vi "ILCDisabledTest.vi"() -> ()   [LabVIEW 2016]
uses:
  Common_RT_HPILC/DataTypes/HPTelemetry.ctl
  Stats.ctl
  Common_RT_Modbus/DataTypes/RxFrame.ctl
  Common_RT_HealthAndStatus/RTHealthAndStatus/RTHealthAndStatus.lvclass
  MyHealthAndStatusReadFIFO/MyHealthAndStatusReadFIFO.lvclass
  D:/Code/Common_RT_FPGA/IReadU32FIFO/IReadU32FIFO.lvclass
  MyHealthAndStatusWriteFIFO/MyHealthAndStatusWriteFIFO.lvclass
  D:/Code/Common_RT_FPGA/IWriteU64FIFO/IWriteU64FIFO.lvclass
  ModbusFactory/ModbusFactory.lvclass
  D:/Code/Common_RT_Modbus/IModbusFactory/IModbusFactory.lvclass
  SubnetFactory/SubnetFactory.lvclass
  Subnet/DataTypes/SubnetSettings.ctl
  Common_RT_HPILC/DataTypes/HPSettings.ctl
  Common_RT_ILC/DataTypes/ILCSettings.ctl
  Common_RT_Modbus/IModbusFactory/IModbusFactory.lvclass
  Common_RT_MTILC/DataTypes/MTSettings.ctl
  Common_RT_MDILC/DataTypes/MDSettings.ctl
  Common_RT_MIILC/DataTypes/MISettings.ctl
  ModbusFactory/ModbusFactory.lvclass/ModbusFactory.ctl
  MyHealthAndStatusWriteFIFO/MyHealthAndStatusWriteFIFO.lvclass/MyHealthAndStatusWriteFIFO.ctl
  MyHealthAndStatusReadFIFO/MyHealthAndStatusReadFIFO.lvclass/MyHealthAndStatusReadFIFO.ctl
  Common_RT_HealthAndStatus/RTHealthAndStatus/RTHealthAndStatus.lvclass/RTHealthAndStatus.ctl
  Subnet/Subnet.lvclass/Subnet.ctl
  Common_RT_HPILC/HPILC/HPILC.lvclass/HPILC.ctl
  <vilib>/Platform/TimedLoop/XDataNode/timing_clust.ctl
  <vilib>/Platform/TimedLoop/XDataNode/nitl_modes.ctl
  <vilib>/Platform/TimedLoop/XDataNode/wakeup.ctl
  Common_RT_MIILC/MIILC/MIILC.lvclass/MIILC.ctl
  Common_RT_MDILC/MDILC/MDILC.lvclass/MDILC.ctl
  Common_RT_MTILC/MTILC/MTILC.lvclass/MTILC.ctl
  <vilib>/FPGAPlugInAG/cRIO-9038/niLvFpga_Open_cRIO-9038.vi
  <vilib>/rvi/interface/common/dynamic/niFpgaDynamicAddResources.vi
  <vilib>/FPGAPlugInAG/Dynamic/niLvFpga_Abort_Dynamic.vi
  <vilib>/FPGAPlugInAG/Dynamic/niLvFpga_Reset_Dynamic.vi
  <vilib>/FPGAPlugInAG/Dynamic/niLvFpga_Run_Dynamic.vi
  <vilib>/Utility/error.llb/Error Cluster From Error Code.vi
  <vilib>/rvi/errors/niLvFpgaAdjustHostInterfaceError.vi
  <vilib>/FPGAPlugInAG/Dynamic/niLvFpga_Close_Dynamic.vi
  <vilib>/rvi/interface/nirviOpenFPGA/nirviOpenFPGA.xnode
  FPGA Bitfiles/modbus1Port.lvbitx
  FPGA/main.vi
  <vilib>/rvi/interface/nirviMethod/nirviMethod.xnode
  <vilib>/Platform/TimedLoop/XDataNode/XDataNode.xnode
  <vilib>/rvi/interface/nirviCloseFPGA/nirviCloseFPGA.xnode
  Subnet/Subnet.lvclass
  Common_RT_ILC/RTILC.lvlib
  Common_RT_HPILC/RTHPILC.lvlib
  Common_RT_HPILC/HPILC/HPILC.lvclass
  <vilib>/rvi/errors/niLvFpgaMergeErrorWithErrorCode.vi
  <vilib>/FPGAPlugInAG/Dynamic/niLvFpga_ReadFifo_Dynamic.vi
  Common_RT_MTILC/MTILC/MTILC.lvclass
  Common_RT_MDILC/MDILC/MDILC.lvclass
  Common_RT_MIILC/MIILC/MIILC.lvclass
  Common_RT_MIILC/RTMIILC.lvlib
  Common_RT_MDILC/RTMDILC.lvlib
  Common_RT_MTILC/RTMTILC.lvlib
  <vilib>/Platform/TimedLoop/XDataNode/XDNodeRunTimeDep.lvlib
  Common_RT_Modbus/RTModbus.lvlib
panel:
  out "Avg Time Delta":dbl
  out "Min Time Delta":i64
  out "Max Time Delta":i64
  out "Timestamp":i64
  out "CRC":T1[](array[typedef]) {"Data" format="%02x"}
  out "Displacement":T2(graph)
  out "Inclination":cluster{"Angle":sgl}(graph)
  out "Temperature":T3(graph)
  out "output cluster":T4={"MinLoopTime"=99999.0, "MaxLoopTime"=-99999.0}
  in  "Steps":i32=1
  out "Loop Time":cluster{u32, "Messages":i32}(graph)
  out "InvalidCRCs":i32
  out "Actuator Telemetry":T5[](array[typedef])
  out "Encoder":T6(graph)
  in  "Stop":bool
  out "Port 1 Status Bits":u64 format="%016b"
  out "error out":errorcluster
  out "Port 1 Frames Received":i64
  out "Port 1 Bytes Received":i64
  out "Port 1 Frames Transmitted":i64
  out "Port 1 Bytes Transmitted":i64
  # "Port 1 = Modbus"
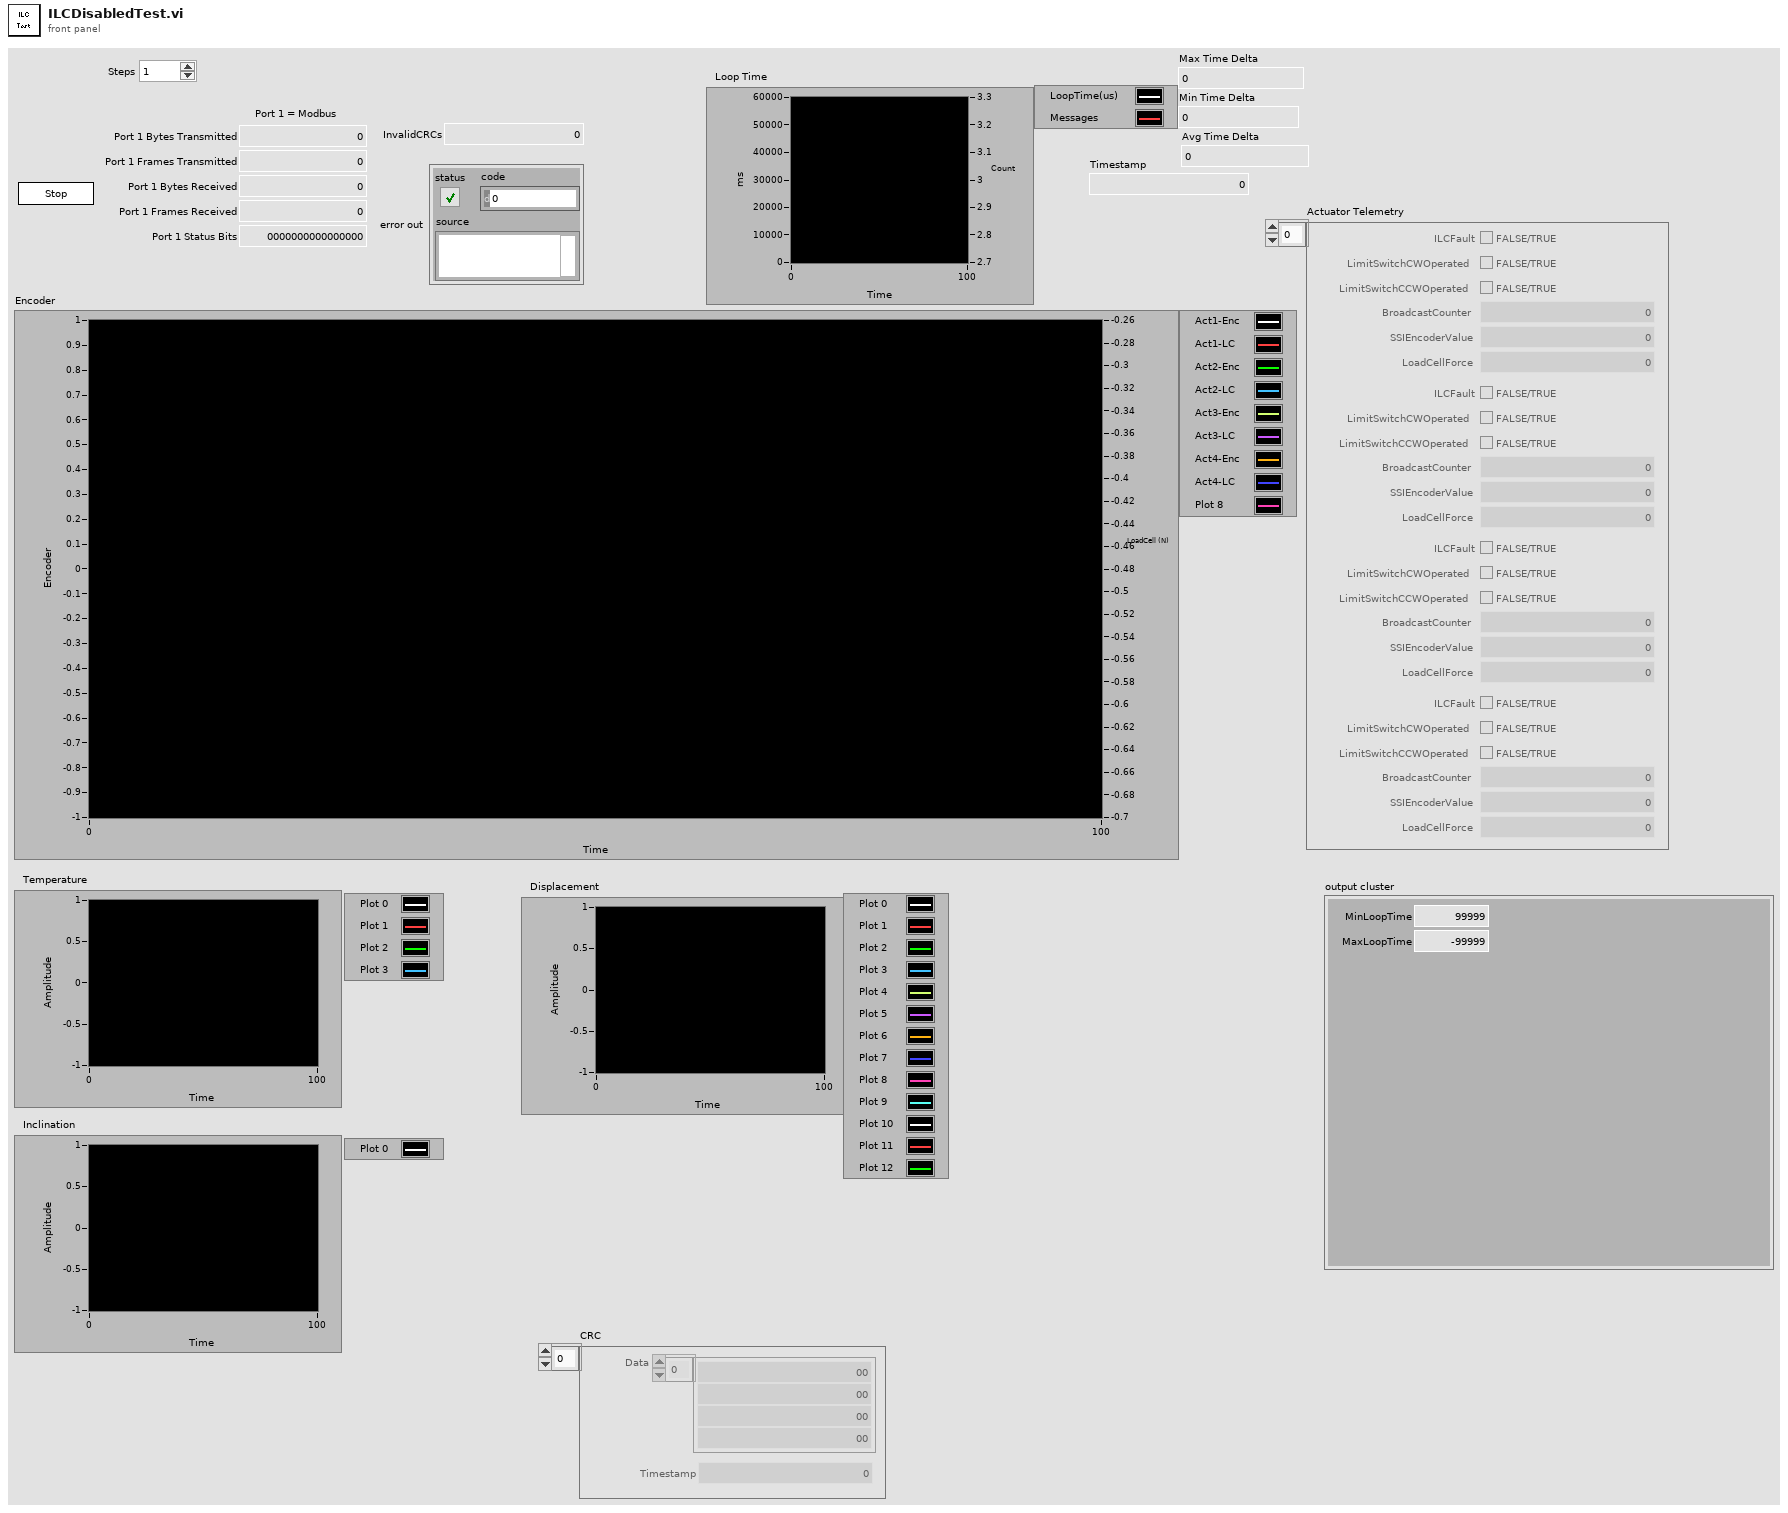
[diagram p1: front panel]
types:
  T1 = typedef "RTModbus.lvlib/RxFrame.ctl" = cluster{"Data":u8[], "Timestamp":u64}
  T2 = cluster{"Displacement1":sgl, "Displacement1":sgl, "Displacement1":sgl, "Displacement1":sgl, "Displacement1":sgl, "Displacement1":sgl}
  T3 = cluster{"Temperature1":sgl, "Temperature1":sgl, "Temperature1":sgl, "Temperature1":sgl}
  T4 = typedef "Stats.ctl" = cluster{"MinLoopTime":dbl, "MaxLoopTime":dbl}
  T5 = typedef "RTHPILC.lvlib/HPTelemetry.ctl" = cluster{"ILCFault":bool, "LimitSwitchCWOperated":bool, "LimitSwitchCCWOperated":bool, "BroadcastCounter":u8, "SSIEncoderValue":i32, "LoadCellForce":sgl}
  T6 = cluster{"[0]":dbl, "[1]":dbl, "[2]":dbl, "[3]":dbl, "[4]":dbl, "[5]":dbl, "[6]":dbl, "[7]":dbl, "[8]":dbl}
  T7 = typedef "RTMIILC.lvlib/MISettings.ctl" = cluster{"ILCSettings":T8, "ID":i16}
  T8 = typedef "RTILC.lvlib/ILCSettings.ctl" = cluster{"Subnet":u8, "Address":u8}
  T9 = typedef "RTMDILC.lvlib/MDSettings.ctl" = cluster{"ILCSettings":T8, "ID":i16}
  T10 = typedef "RTMTILC.lvlib/MTSettings.ctl" = cluster{"ILCSettings":T8, "ID":i16}
  T11 = typedef "RTHPILC.lvlib/HPSettings.ctl" = cluster{"ILCSettings":T8, "ID":i16, "ReferencePosition":i32}
  T12 = enum16{"open", "replace", "create", "open or create", "replace or create", "replace or create with confirmation"}
  T13 = typedef "XDNodeRunTimeDep.lvlib/timing_clust.ctl" = cluster{"Expected End [f-1]":u64, "Actual End [f-1]":u64, "Finished Late? [f-1]":bool, "Expected End [i-1]":u64, "Actual End [i-1]":u64, "Finished Late? [i-1]":bool, "Expected Start [i]":u64, "Actual Start [i]":u64, "Expected Start [f]":u64, "Actual Start [f]":u64, "Source Name":string, "Structure Name":string, "Period":i64, "Deadline":i64, "Offset":i64, "Start":i64, "Priority":i32, "Timeout":i32, "Mode":T14, "Wakeup Reason":T15, "Error":errorcluster, "Source Type":string, "Secondary Source Type":string, "Global End Time":u64, "Global Start Time":u64, "Frame Duration":u64, "Iteration Duration":u64, "Assigned CPU":i32, "I/O Scan Engine Mode":u32}
  T14 = typedef "XDNodeRunTimeDep.lvlib/nitl_modes.ctl" = enum32{"No Change", "Process missed periods, maintain original phase", "Discard missed periods, maintain original phase", "Process missed periods, ignore original phase", "Discard missed periods, ignore original phase"}
  T15 = typedef "XDNodeRunTimeDep.lvlib/wakeup.ctl" = enum32{"Normal", "Aborted", "Asynchronous wakeup", "Timing source error", "Timed loop error", "Timeout"}
  T16 = typedef "SubnetSettings.ctl" = cluster{"HPs":T11[], "ModbusFactory":refnum<class "IModbusFactory.lvclass">, "Port":i32, "MTs":T10[], "MDs":T9[], "MIs":T7[]}
  T17 = typedef "SubnetData.ctl" = cluster{"SubnetConstants":T18, "SubnetCommand":T21, "SubnetTelemetry":T22}
  T18 = typedef "SubnetConstants.ctl" = cluster{"Modbus":refnum<class "IModbus.lvclass">, "HPs":refnum<class "HPILC.lvclass">[], "AddressToActuator":T19[], "MTs":refnum<class "MTILC.lvclass">[], "MDs":refnum<class "MDILC.lvclass">[], "MIs":refnum<class "MIILC.lvclass">[]}
  T19 = typedef "ILCIndexData.ctl" = cluster{"ILCTypes":T20, "Index":i32}
  T20 = typedef "ILCTypes.ctl" = enum16{"Undefined", "SAA", "DAA", "HP", "MT", "MD", "MI"}
  T21 = typedef "SubnetCommand.ctl" = cluster{"BroadcastCounter":u8}
  T22 = typedef "SubnetTelemetry.ctl" = cluster{"BytesTransmitted":u32, "FramesTransmitted":u32, "BytesReceived":u32, "FramesReceived":u32, "TxInternalFIFOOverflow":bool, "InvalidInstruction":bool, "WaitForRxFrameTimeout":bool, "StartBitError":bool, "StopBitError":bool, "RxDataFIFOOverflow":bool}
  T23 = typedef "RTHPILC.lvlib/HPData.ctl" = cluster{"Constants":T24, "Command":T25, "Telemetry":T5, "Responses":T26, "Timings":T28}
  T24 = typedef "RTHPILC.lvlib/HPConstants.ctl" = cluster{"ID":i16, "ReferencePosition":i32}
  T25 = typedef "RTHPILC.lvlib/HPCommand.ctl" = cluster{"Steps":i8}
  T26 = typedef "RTHPILC.lvlib/HPResponses.ctl" = cluster{"StepMotor":T27, "ForceAndStatus":T27}
  T27 = typedef "RTModbus.lvlib/ExceptionCodes.ctl" = u16
  T28 = typedef "RTHPILC.lvlib/HPTimings.ctl" = cluster{"BroadcastStepMotor":u32, "ForceAndStatus":u32, "FreezeSensorValues":u32, "StepMotor":u32}
  T29 = typedef "RTMTILC.lvlib/MTData.ctl" = cluster{"Constants":T30, "Telemetry":T31, "Responses":T32, "Timings":T33}
  T30 = typedef "RTMTILC.lvlib/MTConstants.ctl" = cluster{"ID":i16}
  T31 = typedef "RTMTILC.lvlib/MTTelemetry.ctl" = cluster{"Temperature":sgl[]}
  T32 = typedef "RTMTILC.lvlib/MTResponses.ctl" = cluster{"Temperature":T27}
  T33 = typedef "RTMTILC.lvlib/MTTimings.ctl" = cluster{"Temperature":u32}
  T34 = typedef "RTMDILC.lvlib/MDData.ctl" = cluster{"Constants":T35, "Telemetry":T36, "Responses":T37, "Timings":T38}
  T35 = typedef "RTMDILC.lvlib/MDConstants.ctl" = cluster{"ID":i16}
  T36 = typedef "RTMDILC.lvlib/MDTelemetry.ctl" = cluster{"Displacement":sgl[]}
  T37 = typedef "RTMDILC.lvlib/MDResponses.ctl" = cluster{"Displacement":T27}
  T38 = typedef "RTMDILC.lvlib/MDTimings.ctl" = cluster{"Displacement":u32}
  T39 = typedef "RTMIILC.lvlib/MIData.ctl" = cluster{"Constants":T40, "Telemetry":T41, "Responses":T42, "Timings":T43}
  T40 = typedef "RTMIILC.lvlib/MIConstants.ctl" = cluster{"ID":i16}
  T41 = typedef "RTMIILC.lvlib/MITelemetry.ctl" = cluster{"Angle":sgl}
  T42 = typedef "RTMIILC.lvlib/MIResponses.ctl" = cluster{"Inclination":T27}
  T43 = typedef "RTMIILC.lvlib/MITimings.ctl" = cluster{"Inclination":u32}
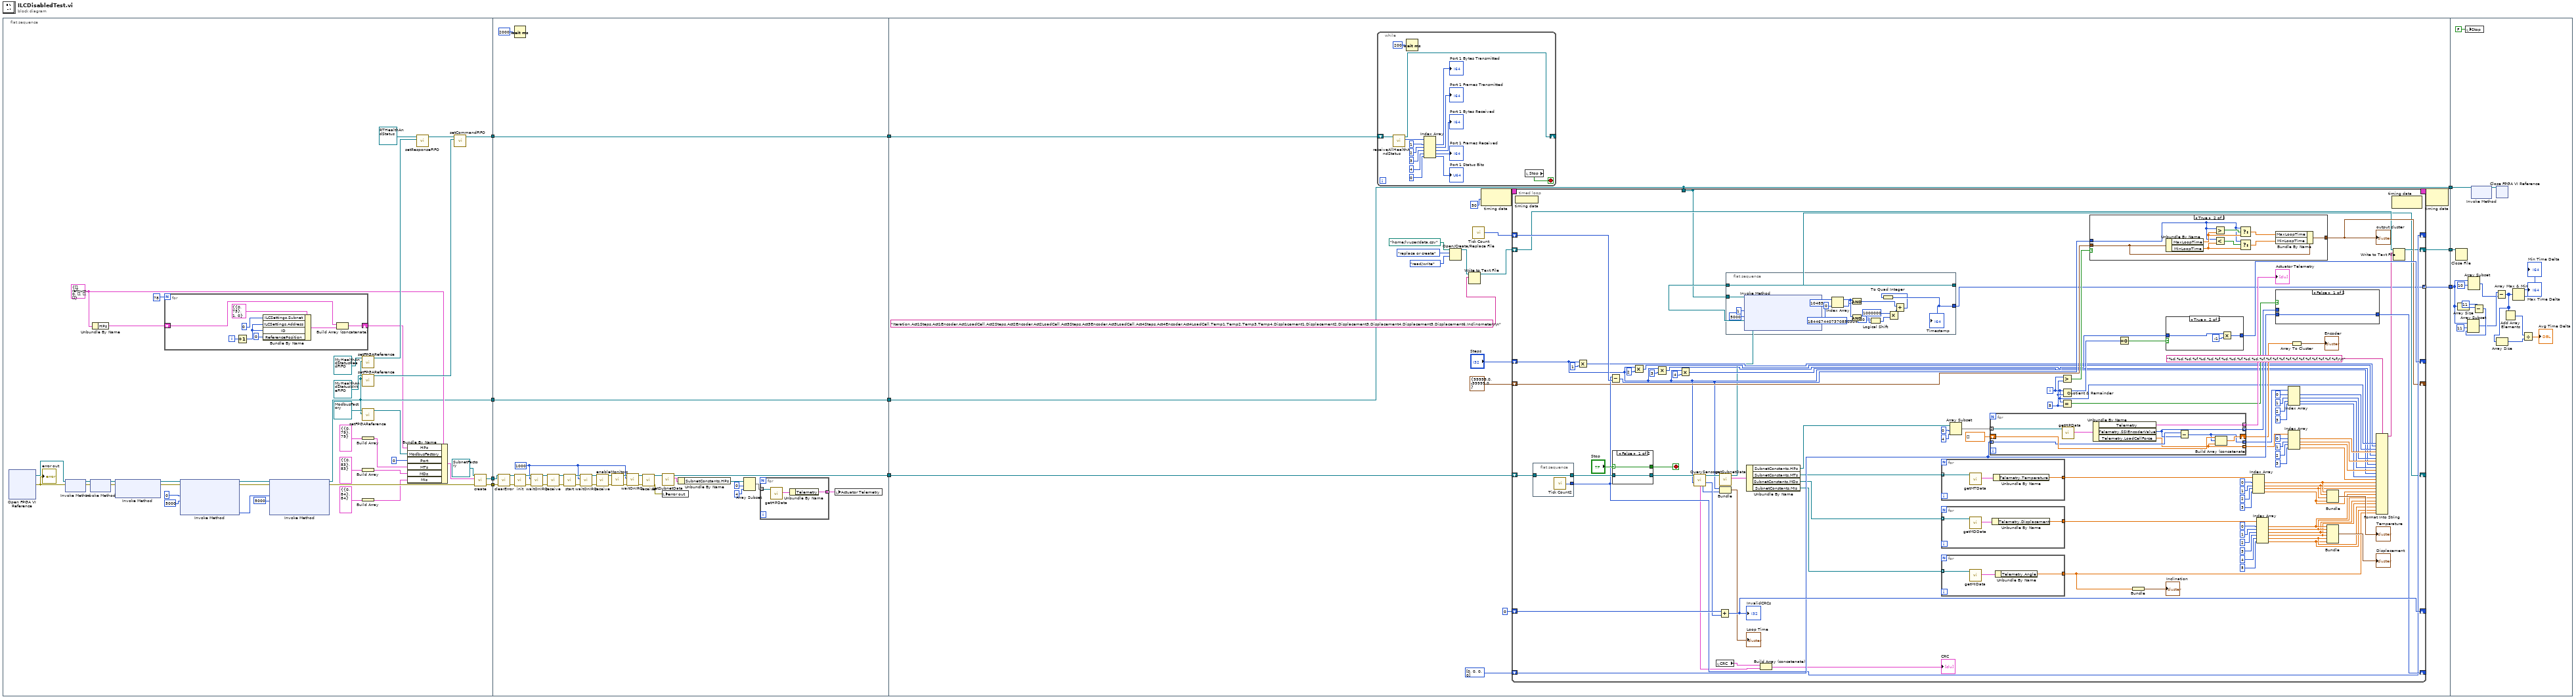
[diagram p0: block diagram]
diagram:
  n1 = flat-sequence {
    tunnel: [w25] -> w10
    tunnel: [w47] -> w7
    tunnel: [w34] -> w5
    tunnel: [w18] -> w3
    tunnel: w10 -> [w91]
    tunnel: [w91] -> w9
    tunnel: w7 -> [w89]
    tunnel: [w89] -> w6
    tunnel: w5 -> [w76]
    tunnel: [w77] -> w4
    tunnel: w3 -> [w68]
    tunnel: w9 -> [w96]
    tunnel: [w96] -> w8
    tunnel: w6 -> [w113]
    tunnel: w4 -> [w112]
    tunnel: [w103] -> w2
    tunnel: [w95] -> w1
    tunnel: w8 -> [w310]
    tunnel: w2 -> [w308]
    tunnel: w1 -> [w307]
    frame #0 {
      w39 = T16 {"HPs"=[], "ModbusFactory"=refnum, "Port"=0, "MTs"=[], "MDs"=[], "MIs"=[]} ("SubnetSettings")
      n2 = xnode "Open FPGA VI Reference"() -> ("FPGA VI Reference Out"=w41:refnum<k20>, "error out"=w20:errorcluster)  [unwired: 2 in]
      "error out" <- w20
      n3 = xnode "Invoke Method"("FPGA VI Reference In"=w41, "error in"=w20) -> ("FPGA VI Reference Out"=w50:refnum<k20>, "error out"=w42:errorcluster)
      n4 = xnode "Invoke Method"("FPGA VI Reference In"=w50, "error in"=w42) -> ("FPGA VI Reference Out"=w27:refnum<k20>, "error out"=w24:errorcluster)
      n5 = Unbundle By Name(w39) -> ("HPs"=w22:T11[])
      n6 = xnode "Invoke Method"("FPGA VI Reference In"=w27, "error in"=w24) -> ("FPGA VI Reference Out"=w26:refnum<k20>, "error out"=w23:errorcluster)  [unwired: 1 in]
      n7 = for {
        N: 78 -> [_]
        shift-right: [w52] -> w21
        shift-left: w22 -> [w53]
        i -> [w57]
        n8 = Increment(x=w57) -> (x+1=w51:i32)
        n9 = Bundle By Name(cluster=T11 {"ILCSettings"={"Subnet"=0, "Address"=73}, "ID"=1, "ReferencePosition"=0} ("HPSettings"), "ILCSettings.Subnet"=u8 0, "ILCSettings.Address"=w51, "ID"=w51, "ReferencePosition"=0) -> (w54:T11)
        n10 = Build Array (concatenate)(w53, w54) -> (w52:T11[])
      }
      n11 = xnode "Invoke Method"("FPGA VI Reference In"=w26, "error in"=w23, "Number of Elements"=u32 0, "Timeout (ms)"=5000) -> ("FPGA VI Reference Out"=w30:refnum<k20>, "error out"=w28:errorcluster, "Elements Remaining"=w31:u32)  [unwired: 1 out]
      n12 = xnode "Invoke Method"("FPGA VI Reference In"=w30, "error in"=w28, "Number of Elements"=w31, "Timeout (ms)"=5000) -> ("FPGA VI Reference Out"=w25:refnum<k20>, "error out"=w19:errorcluster)  [unwired: 2 out]
      n13 = call "setFPGAReference.vi"("FPGAReference"=w25, "MyHealthAndStatusReadFIFO in"=refnum<class "MyHealthAndStatusReadFIFO.lvclass"> refnum ("MyHealthAndStatusReadFIFO.lvclass")) -> ("MyHealthAndStatusReadFIFO out"=w45:refnum<class "MyHealthAndStatusReadFIFO.lvclass">)  [unwired: 9 in]
      n14 = call "setFPGAReference.vi"("FPGAReference"=w25, "MyHealthAndStatusWriteFIFO in"=refnum<class "MyHealthAndStatusWriteFIFO.lvclass"> refnum ("MyHealthAndStatusWriteFIFO.lvclass")) -> ("MyHealthAndStatusWriteFIFO out"=w43:refnum<class "MyHealthAndStatusWriteFIFO.lvclass">)  [unwired: 9 in]
      n15 = call "setFPGAReference.vi"("FPGAReference"=w25, "ModbusFactory in"=refnum<class "ModbusFactory.lvclass"> refnum ("ModbusFactory.lvclass")) -> ("ModbusFactory out"=w37:refnum<class "ModbusFactory.lvclass">)  [unwired: 9 in]
      n16 = Build Array(T10 {"ILCSettings"={"Subnet"=0, "Address"=79}, "ID"=79} ("MTSettings")) -> (w11:T10[])
      n17 = Build Array(T9 {"ILCSettings"={"Subnet"=0, "Address"=83}, "ID"=83} ("MDSettings")) -> (w12:T9[])
      n18 = Build Array(T7 {"ILCSettings"={"Subnet"=0, "Address"=84}, "ID"=84} ("MISettings")) -> (w13:T7[])
      n19 = Bundle By Name(cluster=w39, "HPs"=w21, "ModbusFactory"=w37, "Port"=0, "MTs"=w11, "MDs"=w12, "MIs"=w13) -> (w36:T16)
      n20 = call "setResponseFIFO.vi"("ReadU32FIFO"=w45, "RTHealthAndStatus in"=refnum<class "RTHealthAndStatus.lvclass"> refnum ("RTHealthAndStatus.lvlib:RTHealthAndStatus.lvclass")) -> ("RTHealthAndStatus out"=w48:refnum<class "RTHealthAndStatus.lvclass">)  [unwired: 9 in]
      n21 = call "setCommandFIFO.vi"("WriteU64FIFO"=w43, "RTHealthAndStatus in"=w48) -> ("RTHealthAndStatus out"=w47:refnum<class "RTHealthAndStatus.lvclass">)  [unwired: 9 in]
      n22 = call "create.vi"("error in (no error)"=w19, "SubnetSettings"=w36, "SubnetFactory in"=refnum<class "SubnetFactory.lvclass"> refnum ("SubnetFactory.lvclass")) -> ("error out"=w18:errorcluster, "Subnet"=w34:refnum<class "Subnet.lvclass">)  [unwired: 6 in, 1 out]
    }
    frame #1 {
      w59 = 1000 ("Timeout (ms)")
      n23 = call-dynamic "clearError.vi"("error in (no error)"=w68, "Subnet in"=w76) -> ("error out"=w74:errorcluster, "Subnet out"=w75:refnum<class "Subnet.lvclass">)  [unwired: 8 in]
      n24 = Wait (ms)(milliseconds to wait=u32 2000) -> ()  [unwired: 1 out]
      n25 = call-dynamic "init.vi"("error in (no error)"=w74, "Subnet in"=w75) -> ("error out"=w85:errorcluster, "Subnet out"=w88:refnum<class "Subnet.lvclass">)  [unwired: 8 in]
      n26 = call-dynamic "waitOnIRQ.vi"("error in (no error)"=w85, "Timeout (ms)"=w59, "Subnet in"=w88) -> ("error out"=w86:errorcluster, "Subnet out"=w87:refnum<class "Subnet.lvclass">)  [unwired: 7 in]
      n27 = call-dynamic "receive.vi"("Subnet in"=w87, "error in (no error)"=w86) -> ("Subnet out"=w84:refnum<class "Subnet.lvclass">, "error out"=w82:errorcluster)  [unwired: 8 in, 4 out]
      n28 = call-dynamic "start.vi"("error in (no error)"=w82, "Subnet in"=w84) -> ("error out"=w81:errorcluster, "Subnet out"=w83:refnum<class "Subnet.lvclass">)  [unwired: 8 in]
      n29 = call-dynamic "waitOnIRQ.vi"("error in (no error)"=w81, "Timeout (ms)"=w59, "Subnet in"=w83) -> ("error out"=w79:errorcluster, "Subnet out"=w80:refnum<class "Subnet.lvclass">)  [unwired: 7 in]
      n30 = call-dynamic "receive.vi"("Subnet in"=w80, "error in (no error)"=w79) -> ("Subnet out"=w67:refnum<class "Subnet.lvclass">, "error out"=w64:errorcluster)  [unwired: 8 in, 4 out]
      n31 = call-dynamic "enableMonitors.vi"("error in (no error)"=w64, "Subnet in"=w67) -> ("error out"=w63:errorcluster, "Subnet out"=w66:refnum<class "Subnet.lvclass">)  [unwired: 8 in]
      n32 = call-dynamic "waitOnIRQ.vi"("error in (no error)"=w63, "Timeout (ms)"=w59, "Subnet in"=w66) -> ("error out"=w62:errorcluster, "Subnet out"=w65:refnum<class "Subnet.lvclass">)  [unwired: 7 in]
      n33 = call-dynamic "receive.vi"("Subnet in"=w65, "error in (no error)"=w62) -> ("Subnet out"=w60:refnum<class "Subnet.lvclass">, "error out"=w61:errorcluster)  [unwired: 8 in, 4 out]
      n34 = call "getSubnetData.vi"("Subnet in"=w60) -> ("SubnetData"=w78:T17, "Subnet out"=w77:refnum<class "Subnet.lvclass">)  [unwired: 9 in]
      n35 = local write "error out"(w61) -> ()
      n36 = Unbundle By Name(w78) -> ("SubnetConstants.HPs"=w73:refnum<class "HPILC.lvclass">[])
      n37 = Array Subset(array=w73, index=0, length=4) -> (w70:refnum<class "HPILC.lvclass">[])
      n38 = for {
        tunnel: w70 -> [w94] mode=indexing
        tunnel: [w92] -> w69 mode=indexing
        n39 = call "getHPData.vi"("HardPointActuator in"=w94) -> ("HPData"=w93:T23)  [unwired: 9 in, 1 out]
        n40 = Unbundle By Name(w93) -> ("Telemetry"=w92:T5)
      }
      n41 = local write "Actuator Telemetry"(w69) -> ()
    }
    frame #2 {
      n42 = while {
        shift-right: [w291] -> _
        shift-left: w113 -> [w292]
        stop <- w279 stop-if-true
        n43 = call "receiveAllHealthAndStatus.vi"("RTHealthAndStatus in"=w292) -> ("Data"=w286:u32[], "RTHealthAndStatus out"=w291:refnum<class "RTHealthAndStatus.lvclass">)  [unwired: 8 in, 1 out]
        n44 = Wait (ms)(milliseconds to wait=u32 200) -> ()  [unwired: 1 out]
        n45 = Index Array(array=w286, index #1=1 ("index"), index #2=2 ("index"), index #3=3 ("index"), index #4=4 ("index"), index #5=0 ("index")) -> (element #1=→"Port 1 Bytes Transmitted":u32, element #2=→"Port 1 Frames Transmitted":u32, element #3=→"Port 1 Bytes Received":u32, element #4=→"Port 1 Frames Received":u32, element #5=→"Port 1 Status Bits":u32)
        n46 = local read "Stop"() -> (w279:bool)
      }
      n47 = Open/Create/Replace File(file path (use dialog)=path "/home/lvuser/data.csv", operation (0:open)=T12."replace or create", access (0:read/write)=enum16{"read/write", "read-only", "write-only"}."read/write") -> (refnum out=w102:refnum<file>)  [unwired: 3 in, 2 out]
      n48 = Write to Text File(file (use dialog)=w102, text="Iteration,Act1Steps,Act1Encoder,Act1LoadCell,Act2Steps,Act2Encoder,Act2LoadCell,Act3Steps,Act3Encoder,Act3LoadCell,Act4Steps,Act4Encoder,Act4LoadCell,Temp1,Temp2,Temp3,Temp4,Displacement1,Displacement2,Displacement3,Displacement4,Displacement5,Displacement6,Inclinometer\r\n" ("format string")) -> (refnum out=w101:refnum<file>)  [unwired: 2 in, 2 out]
      n49 = call "Tick Count"() -> ("Tick Count(uSec)"=w110:u32)
      n50 = node-c288(i64 50 ("Period")) -> (w99:T13)
      n51 = timed-loop {
        shift-right: [w116] -> _
        shift-left: w112 -> [w192]
        shift-right: [w200] -> _
        shift-left: "Steps" -> [w159]
        shift-right: [w204] -> _
        shift-left: 0 -> [w205]
        shift-right: [w190] -> _
        shift-left: w110 -> [w203]
        shift-right: [w197] -> _
        shift-left: i32[] [0, 0, 0, 0] -> [w196]
        shift-right: [w183] -> _
        shift-left: T4 {"MinLoopTime"=99999.0, "MaxLoopTime"=-99999.0} ("Stats") -> [w184]
        shift-right: [w118] -> w103
        shift-left: w101 -> [w119]
        timing: w99 -> [_]
        timing-out: [_] -> w98
        tunnel: [w115] -> _
        tunnel: w96 -> [w115]
        tunnel: [w114] -> w95 mode=indexing
        i -> [w149]
        stop <- w214 stop-if-true
        w185 = 5 ("y")
        n52 = node-c288() -> ()  [unwired: 1 in]
        n53 = flat-sequence {
          tunnel: w192 -> [w255]
          tunnel: [w255] -> w191
          tunnel: [w254] -> w190
          frame #0 {
            n54 = call "Tick Count2"() -> ("Tick Count(uSec)"=w254:u32)
          }
        }
        n55 = Multiply(x=w159, y=1) -> (x*y=w148:i32)
        n56 = Subtract(x=w190, y=w203) -> (x-y=w182:u32)
        n57 = case shown="False" "Stop" {
          selector: "Stop" -> [w271 w273]
          tunnel: [w271 w273] -> w214
          tunnel: w191 -> [w272 w274]
          tunnel: [w272 w274] -> w213
          frame False {
          }
          frame True {
          }
        }
        n58 = Multiply(x=w159, y=2) -> (x*y=w140:i32)
        n59 = Multiply(x=w159, y=3) -> (x*y=w137:i32)
        n60 = Multiply(x=w159, y=4) -> (x*y=w134:i32)
        n61 = call "QuerySensors.vi"("Subnet in"=w213, "Steps"=w159) -> ("Subnet out"=w211:refnum<class "Subnet.lvclass">, "InvalidCRC"=w194:i32, "CRCIssues"=w162:T1[], "Messages"=w193:i32)  [unwired: 7 in, 3 out]
        n62 = local read "CRC"() -> (w163:T1[])
        n63 = Add(x=w205, y=w194) -> (x+y=w204:i32)
        "InvalidCRCs" <- w204
        n64 = Bundle(w182, "Messages"=w193) -> (→"Loop Time":cluster{u32, "Messages":i32})  [unwired: 1 in]
        n65 = call "getSubnetData.vi"("Subnet in"=w211) -> ("SubnetData"=w212:T17, "Subnet out"=w117:refnum<class "Subnet.lvclass">)  [unwired: 9 in]
        n66 = flat-sequence {
          tunnel: w117 -> [w232]
          tunnel: [w232] -> w116
          tunnel: w115 -> [w231]
          tunnel: [w226] -> w114
          frame #0 {
            n67 = xnode "Invoke Method"("FPGA VI Reference In"=w231, "Number of Elements"=u32 1, "Timeout (ms)"=5000) -> ("Data"=w228:u64[])  [unwired: 1 in, 3 out]
            n68 = Index Array(array=w228, index=0) -> (element=w225:u64)
            n69 = And(x=w225, y=u64 1048575) -> (x .and. y?=w217:u64)
            n70 = And(x=w225, y=u64 18446744073708503040) -> (x .and. y?=w222:u64)
            n71 = Logical Shift(y=i16 -20, x=w222) -> (x << y=w220:u64)
            n72 = Multiply(x=u64 1000000, y=w220) -> (x*y=w218:u64)
            n73 = Add(x=w217, y=w218) -> (x+y=w216:u64)
            n74 = To Quad Integer(1:w216) -> (0:w226:i64)
            "Timestamp" <- w226
          }
        }
        n75 = Unbundle By Name(w212) -> ("SubnetConstants.HPs"=w208:refnum<class "HPILC.lvclass">[], "SubnetConstants.MTs"=w181:refnum<class "MTILC.lvclass">[], "SubnetConstants.MDs"=w180:refnum<class "MDILC.lvclass">[], "SubnetConstants.MIs"=w179:refnum<class "MIILC.lvclass">[])
        n76 = Build Array (concatenate)(w163, w162) -> (→"CRC":T1[])
        n77 = for {
          tunnel: w181 -> [w243] mode=indexing
          tunnel: [w241] -> w178
          n78 = call "getMTData.vi"("MTILC in"=w243) -> ("MTData"=w242:T29)  [unwired: 9 in, 1 out]
          n79 = Unbundle By Name(w242) -> ("Telemetry.Temperature"=w241:sgl[])
        }
        n80 = for {
          tunnel: w180 -> [w239] mode=indexing
          tunnel: [w238] -> w171
          n81 = call "getMDData.vi"("MDILC in"=w239) -> ("MDData"=w240:T34)  [unwired: 9 in, 1 out]
          n82 = Unbundle By Name(w240) -> ("Telemetry.Displacement"=w238:sgl[])
        }
        n83 = for {
          tunnel: w179 -> [w237] mode=indexing
          tunnel: [w235] -> w121
          n84 = call "getMIData.vi"("MIILC in"=w237) -> ("MIData"=w236:T39)  [unwired: 9 in, 1 out]
          n85 = Unbundle By Name(w236) -> ("Telemetry.Angle"=w235:sgl)
        }
        n86 = Array Subset(array=w208, index=0, length=4) -> (w207:refnum<class "HPILC.lvclass">[])
        n87 = for {
          tunnel: w207 -> [w270] mode=indexing
          shift-right: [w267] -> w189
          shift-left: dbl[] [] -> [w268]
          tunnel: [w266] -> w199 mode=indexing
          tunnel: [w264] -> w198 mode=indexing
          tunnel: w196 -> [w265] mode=indexing
          tunnel: [w263] -> w154 mode=indexing
          tunnel: [w262] -> w146 mode=indexing
          n88 = call "getHPData.vi"("HardPointActuator in"=w270) -> ("HPData"=w269:T23)  [unwired: 9 in, 1 out]
          n89 = Unbundle By Name(w269) -> ("Telemetry"=w266:T5, "Telemetry.SSIEncoderValue"=w264:i32, "Telemetry.LoadCellForce"=w262:sgl)
          n90 = Subtract(x=w265, y=w264) -> (x-y=w263:i32)
          n91 = Build Array (concatenate)(w268, w263, w262) -> (w267:dbl[])
        }
        "Actuator Telemetry" <- w199
        n92 = Greater?(x=w149, y=w185) -> (0:w186:bool)
        n93 = Equal?(x=w149, y=w185) -> (x = y?=w195:bool)
        n94 = Quotient & Remainder(x=w149, y=w185) -> (x-y*floor(x/y)=w202:i32)  [unwired: 1 out]
        n95 = case shown="True" w186 {
          tunnel: w184 -> [w244 w253]
          tunnel: [w244 w252] -> w183
          tunnel: w182 -> [_ w245]
          frame False {
          }
          frame True {
            n96 = Unbundle By Name(w253) -> ("MaxLoopTime"=w247:dbl, "MinLoopTime"=w246:dbl)
            n97 = Greater?(x=w245, y=w247) -> (0:w250:bool)
            n98 = Less?(x=w245, y=w246) -> (x < y?=w251:bool)
            n99 = Select(t=w245, s=w250, f=w247) -> (s? t:f=w249:dbl)
            n100 = Select(t=w245, s=w251, f=w246) -> (s? t:f=w248:dbl)
            n101 = Bundle By Name(cluster=w253, "MaxLoopTime"=w249, "MinLoopTime"=w248) -> (w252:T4)
          }
        }
        "output cluster" <- w183
        n102 = Equal To 0?(x=w202) -> (x = 0?=w201:bool)
        n103 = Bundle("Angle"=w121) -> (→"Inclination":cluster{"Angle":sgl})  [unwired: 1 in]
        n104 = case shown="True" w201 {
          tunnel: w159 -> [w258 w260]
          tunnel: [w258 w259] -> w200
          frame False {
          }
          frame True {
            n105 = Multiply(x=w260, y=-1) -> (x*y=w259:i32)
          }
        }
        n106 = Index Array(array=w178, index #1=0 ("index"), index #2=1 ("index"), index #3=2 ("index"), index #4=3 ("index")) -> (element #1=w131:sgl, element #2=w130:sgl, element #3=w129:sgl, element #4=w128:sgl)
        n107 = Index Array(array=w171, index #1=0 ("index"), index #2=1 ("index"), index #3=2 ("index"), index #4=3 ("index"), index #5=4 ("index"), index #6=5 ("index")) -> (element #1=w127:sgl, element #2=w126:sgl, element #3=w125:sgl, element #4=w124:sgl, element #5=w123:sgl, element #6=w122:sgl)
        n108 = case shown="False" w195 {
          tunnel: w198 -> [_ w257]
          tunnel: [w256 w257] -> w197
          tunnel: w196 -> [w256 _]
          frame False {
          }
          frame True {
          }
        }
        n109 = Index Array(array=w154, index #1=0 ("index"), index #2=1 ("index"), index #3=2 ("index"), index #4=3 ("index")) -> (element #1=w147:i32, element #2=w139:i32, element #3=w136:i32, element #4=w133:i32)
        n110 = Index Array(array=w146, index #1=0 ("index"), index #2=1 ("index"), index #3=2 ("index"), index #4=3 ("index")) -> (element #1=w141:sgl, element #2=w138:sgl, element #3=w135:sgl, element #4=w132:sgl)
        n111 = Array To Cluster(array=w189) -> (cluster=→"Encoder":T6)
        n112 = Bundle("Displacement1"=w127, "Displacement1"=w126, "Displacement1"=w125, "Displacement1"=w124, "Displacement1"=w123, "Displacement1"=w122) -> (→"Displacement":T2)  [unwired: 1 in]
        n113 = Bundle("Temperature1"=w131, "Temperature1"=w130, "Temperature1"=w129, "Temperature1"=w128) -> (→"Temperature":T3)  [unwired: 1 in]
        n114 = Format Into String(format string="%d,%d,%d,%f,%d,%d,%f,%d,%d,%f,%d,%d,%f,%f,%f,%f,%f,%f,%f,%f,%f,%f,%f,%f\r\n", w149, w148, w147, w141, w140, w139, w138, w137, w136, w135, w134, w133, w132, w131, w130, w129, w128, w127, w126, w125, w124, w123, w122, w121) -> (resulting string=w120:string)  [unwired: 2 in, 1 out]
        n115 = node-c288() -> ()  [unwired: 1 in, 1 out]
        n116 = Write to Text File(file (use dialog)=w119, text=w120) -> (refnum out=w118:refnum<file>)  [unwired: 2 in, 2 out]
      }
      n117 = node-c288(w98) -> ()  [unwired: 1 out]
    }
    frame #3 {
      n118 = Close File(refnum=w308) -> ()  [unwired: 1 in, 2 out]
      n119 = Array Size(array=w307) -> (size(s)=w306:i32)
      n120 = local write "Stop"(FALSE ("Stop")) -> ()
      n121 = Array Subset(array=w307, index=10) -> (w301:i64[])  [unwired: 1 in]
      n122 = xnode "Invoke Method"("FPGA VI Reference In"=w310) -> ("FPGA VI Reference Out"=w311:refnum<k20>)  [unwired: 1 in, 1 out]
      n123 = Subtract(x=w306, y=11) -> (x-y=w304:i32)
      n124 = Array Subset(array=w307, index=11, length=w304) -> (w302:i64[])
      n125 = Subtract(x=w302, y=w301) -> (x-y=w298:i64[])
      n126 = xnode "Close FPGA VI Reference"("FPGA VI Reference In"=w311) -> ()  [unwired: 1 in, 1 out]
      n127 = Array Size(array=w298) -> (size(s)=w296:i32)
      n128 = Add Array Elements(numeric array=w298) -> (sum=w297:i64)
      n129 = Array Max & Min(array=w298) -> (max value=→"Max Time Delta":i64, min value=→"Min Time Delta":i64)  [unwired: 2 out]
      n130 = Divide(x=w297, y=w296) -> (x/y=→"Avg Time Delta":dbl)
    }
  }
